vi "_wait_for_OPC.vi"(5 "Timeout in (0 = OPC timeout)":i32, 7 "Attribute":T1={"Identifier"="", "Descriptive Name"="", "Data Type"=enum."Integer 32", "Command"="", "Access"=enum."Read/Write", "Range Table"="", "Read Callback"="", "Write Callback"="", "Supported Models"="", "Instrument Options"="", "Index"=0, "OPC Wait"=FALSE, "No Status Check"=FALSE, "Cache Only"=FALSE}, 8 "error in":errorcluster caption="error in (no error)", 11 "VISA resource name":refnum<visa-resource-name>) -> (0 "error out":errorcluster, 3 "VISA resource name out":refnum<visa-resource-name>)   [LabVIEW 2020, in "Rohde&Schwarz RTx Oscilloscopes.lvlib" / "rsidr_core.lvlib"]
uses:
  rsidr_core.lvlib
  type_Attribute.ctl
  type_Attribute_Data_Type.ctl
  type_ReadWriteAccess.ctl
  type_Error_Codes.ctl
  Select Event Type.ctl
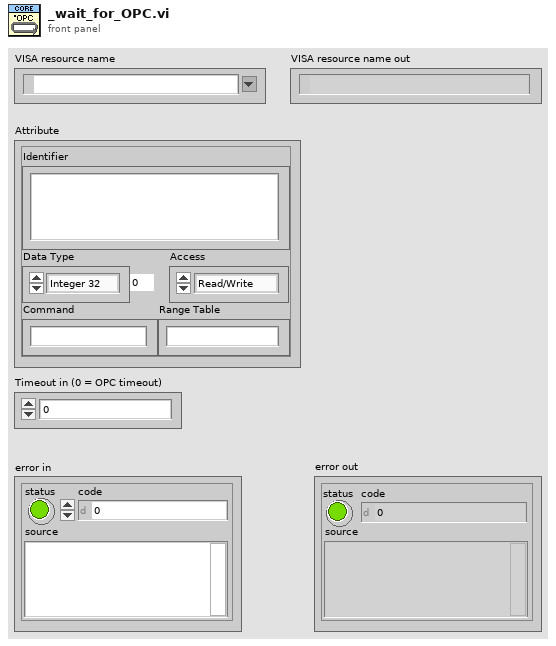
[diagram p1: front panel]
types:
  T1 = typedef "Rohde&Schwarz RTx Oscilloscopes.lvlib/rsidr_core.lvlib/type_Attribute.ctl" = cluster{"Identifier":string, "Descriptive Name":string, "Data Type":T2, "Command":string, "Access":T3, "Range Table":string, "Read Callback":string, "Write Callback":string, "Supported Models":string, "Instrument Options":string, "Index":i32, "OPC Wait":bool, "No Status Check":bool, "Cache Only":bool}
  T2 = typedef "Rohde&Schwarz RTx Oscilloscopes.lvlib/rsidr_core.lvlib/type_Attribute_Data_Type.ctl" = enum16{"Integer 32", "Double", "String", "Boolean", "None", "Integer 64", "RawString"}
  T3 = typedef "Rohde&Schwarz RTx Oscilloscopes.lvlib/rsidr_core.lvlib/type_ReadWriteAccess.ctl" = enum16{"Read Only", "Write Only", "Read/Write"}
  T4 = typedef "Rohde&Schwarz RTx Oscilloscopes.lvlib/rsidr_core.lvlib/type_Error_Codes.ctl" = enum16{"No_error", "VISA_err_ResourceNotFound", "VISA_err_Timeout", "VISA_warn_MoreDataAvailable", "RS_err_MissingCallback", "RS_err_InvalidAttribute", "RS_err_InvalidValue", "RS_err_UnknownResource", "RS_err_AlreadyInitialized", "RS_err_InstrumentStatus", "RS_err_BadRepCapName", "RS_err_TypesMismatch", "RS_err_ValueNotSupported", "RS_err_InvalidRngTable", "RS_err_IDqueryFail", "RS_err_UnexpResponse", "VISA_warn_ConfigNotLoaded", "RS_err_AttributeNotReadable", "RS_err_AttributeNotWritable", "RS_err_InstrumentType", "RS_err_InstrumentOption", "VISA_err_InvalidSize", "RS_err_ReliabilityIndicator", "VISA_warn_UnknownStatus", "VISA_warn_TermCharRead", "VISA_err_IO_error", "RS_err_FunctionNotSupported", "VISA_warn_QueueEmpty"}
  T5 = enum16{"Check error", "Don't check error", "Check error from Session"}
  T6 = typedef "Rohde&Schwarz RTx Oscilloscopes.lvlib/rsidr_core.lvlib/type_Session_Data.ctl" = cluster{"IDN string":string, "Instrument FW":string, "Instr type":string, "Instr type for err. msg.":string, "Installed Options":string[], "Ignore Error Messages":string, "Logging params":variant, "OPC Timeout":i32, "VISA Timeout":i32, "STB Poll VISA Timeout":i32, "Additional Flags":i32, "Wait Before Read":i32, "Wait Before Write":i32, "Option String Flags":i32, "IO Segment Size":i64, "VISA Access Mode":T7, "Interface Type":T8, "OPC Wait Mode":T9, "Bin Float Number  Format":T10, "Bin Integer Number Format":T11, "Simulate":bool, "VXIcapable":bool, "Duplicate Session":bool, "Add LF to Write":bool, "Logging":bool, "Fast Sweep":bool, "Query Instrument Status":bool, "Check Range":bool, "Check Options":bool, "OPC-sync Attr Writes":bool, "OPC-sync Attr Queries":bool}
  T7 = typedef "Rohde&Schwarz RTx Oscilloscopes.lvlib/rsidr_core.lvlib/type_VisaAccessMode.ctl" = u16
  T8 = typedef "Rohde&Schwarz RTx Oscilloscopes.lvlib/rsidr_core.lvlib/type_InterfaceType.ctl" = enum16{"Unknown", "GPIB", "VXI", "GPIB_VXI", "ASRL", "PXI", "TCPIP", "USB", "SOCKET"}
  T9 = typedef "Rohde&Schwarz RTx Oscilloscopes.lvlib/rsidr_core.lvlib/type_OPC_Wait_Mode.ctl" = enum16{"STBpolling", "STBpollingSlow", "STBpollingSuperSlow", "ServiceRequest", "OPCquery"}
  T10 = typedef "Rohde&Schwarz RTx Oscilloscopes.lvlib/rsidr_core.lvlib/type_Binary_Float_Number_Format.ctl" = enum16{"Float_4_Bytes_Swapped", "Float_4_Bytes", "Double_8_Bytes_Swapped", "Double_8_Bytes"}
  T11 = typedef "Rohde&Schwarz RTx Oscilloscopes.lvlib/rsidr_core.lvlib/type_Binary_Integer_Number_Format.ctl" = enum16{"Int32_4_Bytes_Swapped", "Int32_4 Bytes", "Int16_2_Bytes_Swapped", "Int16_2_Bytes"}
  T12 = typedef "Select Event Type.ctl" = u32
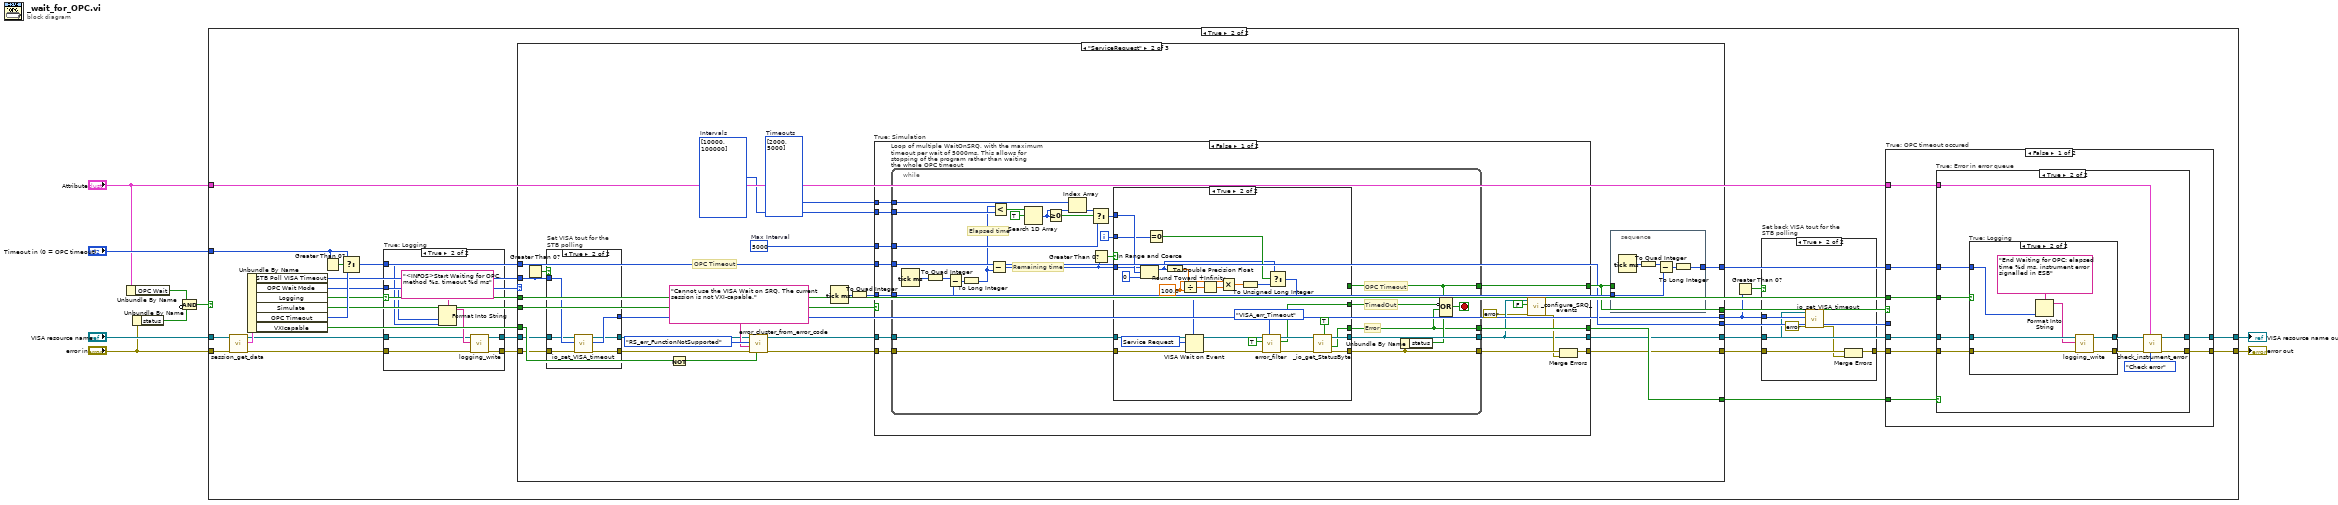
[diagram p0: block diagram]
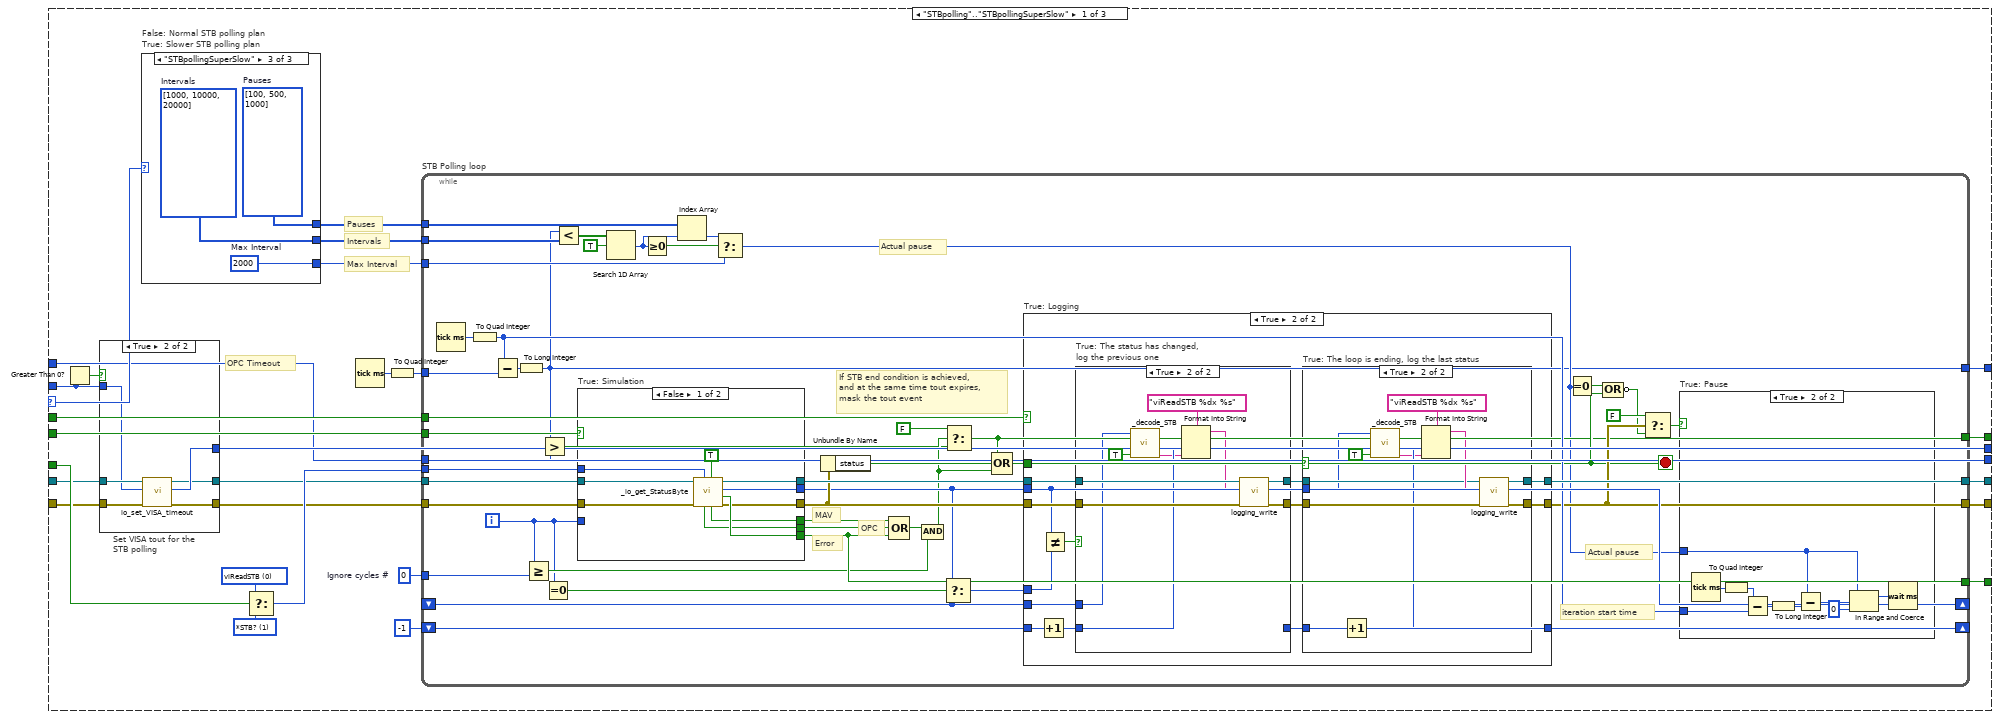
[diagram p5: hidden frame]
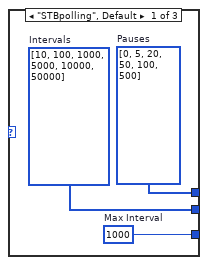
[diagram p7: hidden frame]
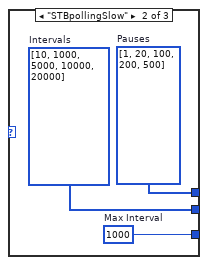
[diagram p8: hidden frame]
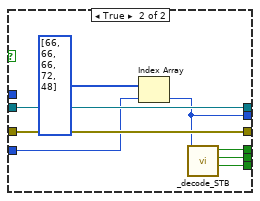
[diagram p10: hidden frame]
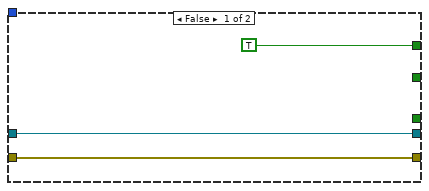
[diagram p15: hidden frame]
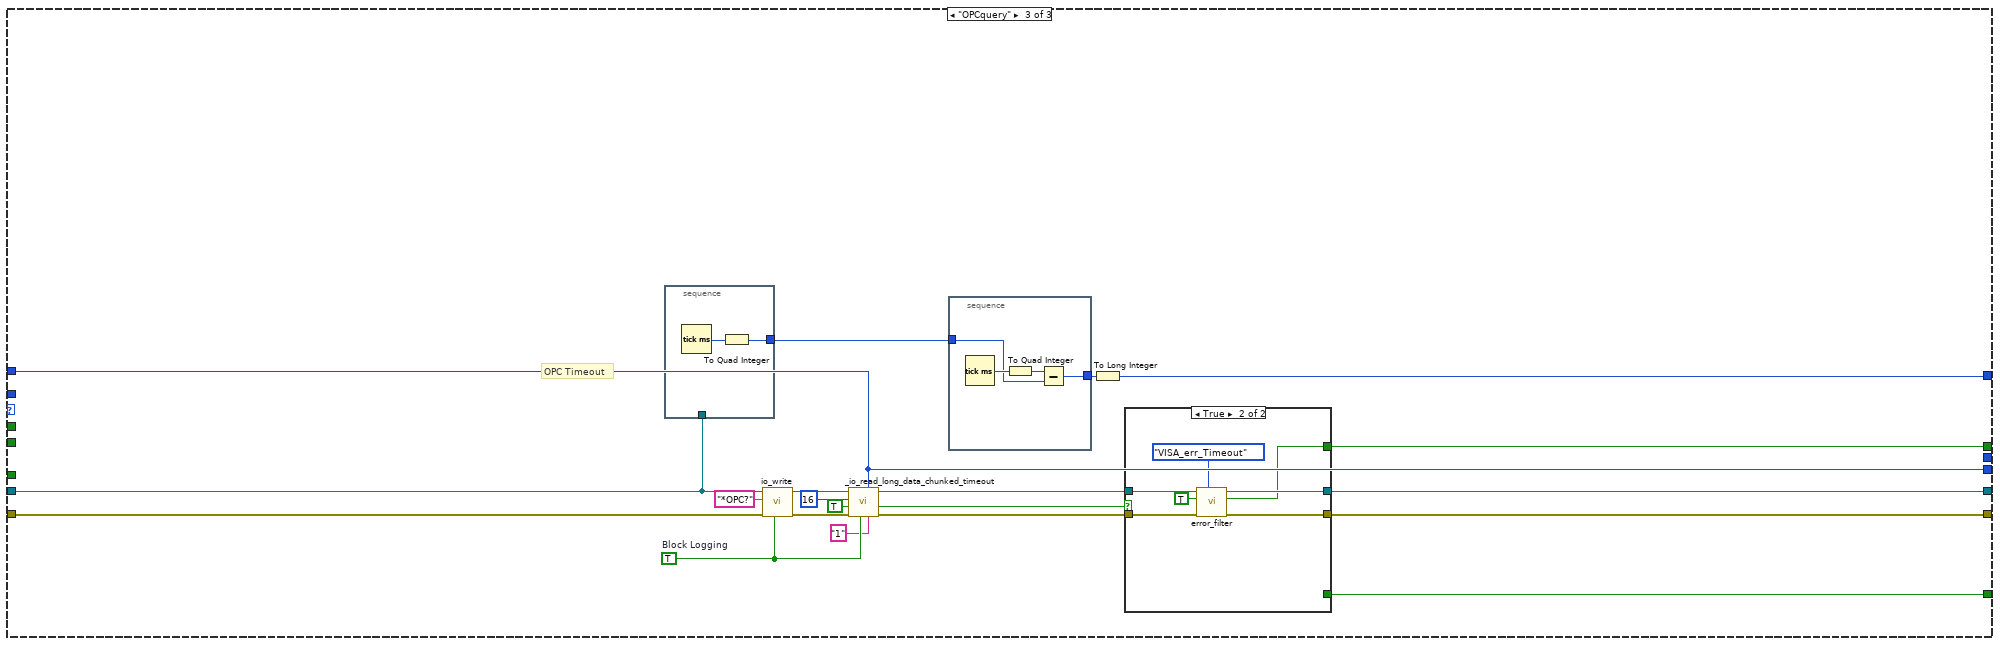
[diagram p17: hidden frame]
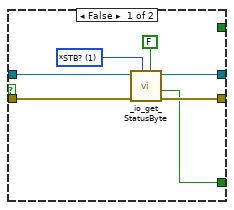
[diagram p18: hidden frame]
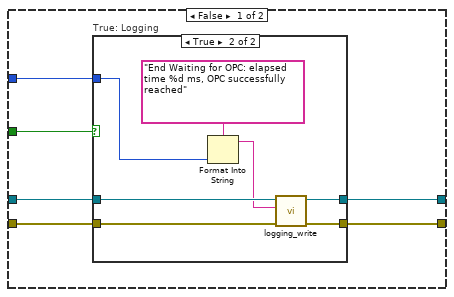
[diagram p19: hidden frame]
diagram:
  n1 = Unbundle By Name("Attribute") -> ("OPC Wait"=w2:bool)
  n2 = Unbundle By Name("error in") -> ("status"=w3:bool)
  n3 = Compound Arithmetic op=AND(w2, invert w3) -> (w1:bool)
  n4 = case shown="True" w1 {
    tunnel: "VISA resource name" -> [w11 w39]
    tunnel: "error in" -> [w10 w38]
    tunnel: [w11 w34] -> w8
    tunnel: [w10 w33] -> w9
    tunnel: "Timeout in (0 = OPC timeout)" -> [_ w27]
    tunnel: "Attribute" -> [_ w32]
    frame False {
    }
    frame True {
      n5 = call "session_get_data.vi"("error in"=w38, "VISA resource name"=w39) -> ("error out"=w25:errorcluster, "Session User Data out"=w37:T6, "VISA resource name out"=w24:refnum<visa-resource-name>)  [unwired: 6 in, 1 out]
      n6 = Unbundle By Name(w37) -> ("STB Poll VISA Timeout"=w19:i32, "OPC Wait Mode"=w20:T9, "Logging"=w21:bool, "Simulate"=w13:bool, "OPC Timeout"=w26:i32, "VXIcapable"=w30:bool)
      n7 = Greater Than 0?(x=w27) -> (x > 0?=w28:bool)
      n8 = Select(t=w27, s=w28, f=w26) -> (s? t:f=w12:i32)
      n9 = case "True: Logging" shown="True" w21 {
        tunnel: [w48 w52] -> w23
        tunnel: [w47 w51] -> w22
        tunnel: w25 -> [w48 w54]
        tunnel: w24 -> [w47 w53]
        tunnel: w20 -> [_ w50]
        tunnel: w12 -> [_ w49]
        frame False {
        }
        frame True {
          n10 = Format Into String(format string="<INFOS>Start Waiting for OPC, method %s, timeout %d ms", w50, w49) -> (resulting string=w56:string)  [unwired: 2 in, 1 out]
          n11 = call "logging_write.vi"("error in"=w54, "String to write"=w56, "VISA resource name"=w53) -> ("error out"=w52:errorcluster, "VISA resource name out"=w51:refnum<visa-resource-name>)  [unwired: 7 in]
        }
      }
      n12 = case shown="\"ServiceRequest\"" w20 {
        selector: w20 -> [w74 _ _]
        tunnel: w22 -> [w64 w226 w341]
        tunnel: [w82 w235 w333] -> w36
        tunnel: [w60 w222 w336] -> w16
        tunnel: [w81 w232 w331] -> w35
        tunnel: w13 -> [w79 w221 _]
        tunnel: w21 -> [w78 _ _]
        tunnel: [w77 w233 w335] -> w31
        tunnel: w23 -> [w65 w227 w348]
        tunnel: [w59 w219 w337] -> w18
        tunnel: w30 -> [w68 w242 _]
        tunnel: [w57 w223 w332] -> w29
        tunnel: w12 -> [w57 w223 w332]
        tunnel: w19 -> [w61 w218 _]
        tunnel: [w58 w220 _] -> w15
        frame "STBpolling".."STBpollingSuperSlow" {
          w69 = u16 1 items=["viReadSTB", "*STB?"] ("Method (viReadSTB)")
          w70 = u16 0 items=["viReadSTB", "*STB?"] ("Method (viReadSTB)")
          w76 = 0  # Ignore cycles #
          # "OPC Timeout"
          # "Pauses"
          # "Intervals"
          # "Max Interval"
          n13 = Greater Than 0?(x=w61) -> (x > 0?=w66:bool)
          n14 = case "Set VISA tout for the\nSTB polling" shown="True" w66 {
            tunnel: w65 -> [w84 w90]
            tunnel: w64 -> [w85 w89]
            tunnel: [w84 w88] -> w63
            tunnel: [w85 w87] -> w62
            tunnel: [_ w91] -> w58
            tunnel: w61 -> [_ w86]
            frame False {
            }
            frame True {
              n15 = call "io_set_VISA_timeout.vi"("error in"=w90, "VISA Timeout"=w86, "VISA resource name"=w89) -> ("error out"=w88:errorcluster, "Old VISA Timeout"=w91:u32, "VISA resource name out"=w87:refnum<visa-resource-name>)  [unwired: 6 in]
            }
          }
          n16 = case "False: Normal STB polling plan\nTrue: Slower STB polling plan" shown="\"STBpollingSuperSlow\"" w74 {
            tunnel: [w92 w95 w98] -> w72
            tunnel: [w94 w97 w100] -> w71
            tunnel: [w93 w96 w99] -> w73
            frame "STBpolling", Default {
              w93 = 1000  # Max Interval
              w92 = i32[] [0, 5, 20, 50, 100, 500]  # Pauses
              w94 = i32[] [10, 100, 1000, 5000, 10000, 50000]  # Intervals
            }
            frame "STBpollingSlow" {
              w96 = 1000  # Max Interval
              w95 = i32[] [1, 20, 100, 200, 500]  # Pauses
              w97 = i32[] [10, 1000, 5000, 10000, 20000]  # Intervals
            }
            frame "STBpollingSuperSlow" {
              w99 = 2000  # Max Interval
              w98 = i32[] [100, 500, 1000]  # Pauses
              w100 = i32[] [1000, 10000, 20000]  # Intervals
            }
          }
          n17 = Select(t=w70, s=w68, f=w69) -> (s? t:f=w67:u16)
          n18 = Tick Count (ms)() -> (millisecond timer value=w83:u32)
          n19 = To Quad Integer(1:w83) -> (0:w75:i64)
          n20 = while "STB Polling loop" {
            tunnel: [w114] -> w77
            tunnel: w75 -> [w147]
            tunnel: w57 -> [w119]
            tunnel: [w138] -> w60
            tunnel: w62 -> [w144]
            tunnel: [w143] -> w82
            tunnel: [w101] -> w81
            shift-right: [w132] -> _
            shift-left: _ -> [w131]
            tunnel: w78 -> [w130]
            shift-right: [w136] -> _
            shift-left: -1 -> [w137]
            tunnel: w79 -> [w134]
            tunnel: w76 -> [w133]
            tunnel: w67 -> [w128]
            tunnel: w63 -> [w121]
            tunnel: [w120] -> w59
            tunnel: w73 -> [w104]
            tunnel: w72 -> [w105]
            tunnel: w71 -> [w106]
            i -> [w127]
            stop <- w117 stop-if-true
            # "Actual pause"
            # "iteration start time"
            # "Actual pause"
            # "If STB end condition is achieved,\nand at the same time tout expires,\nmask the tout event"
            # "OPC"
            # "Error"
            # "MAV"
            n21 = Tick Count (ms)() -> (millisecond timer value=w125:u32)
            n22 = To Quad Integer(1:w125) -> (0:w122:i64)
            n23 = Subtract(x=w122, y=w147) -> (x-y=w107:i64)
            n24 = To Long Integer(number=w107) -> (32bit integer=w101:i32)
            n25 = Greater Or Equal?(x=w127, y=w133) -> (x >= y?=w142:bool)
            n26 = Greater?(x=w101, y=w119) -> (0:w113:bool)
            n27 = Equal To 0?(x=w127) -> (x = 0?=w126:bool)
            n28 = Less?(x=w101, y=w106) -> (x < y?=w111:bool[])
            n29 = case "True: Simulation" shown="False" w134 {
              tunnel: w121 -> [w166 w173]
              tunnel: w144 -> [w165 w174]
              tunnel: [w164 w169] -> w143
              tunnel: [w163 w171] -> w141
              tunnel: [w162 w170] -> w140
              tunnel: [w161 w174] -> w139
              tunnel: [w160 w167] -> w132
              tunnel: [w159 w173] -> w135
              tunnel: w127 -> [_ w172]
              tunnel: w128 -> [w158 _]
              frame False {
                n30 = call "_io_get_StatusByte.vi"("Block Setting of VISA Timeout for viReadSTB"=TRUE, "Method (viReadSTB)"=w158, "error in"=w166, "VISA resource name"=w165) -> ("error out"=w159:errorcluster, "Error"=w164:bool, "STB returned"=w160:u16, "VISA resource name out"=w161:refnum<visa-resource-name>, "MAV"=w162:bool, "OPC (ESB)"=w163:bool)  [unwired: 2 in]
              }
              frame True {
                n31 = Index Array(array=u16[] [66, 66, 66, 72, 48], index=w172) -> (element=w167:u16)
                n32 = call "_decode_STB.vi"("STB in"=w167) -> ("Error"=w169:bool, "OPC (ESB)"=w171:bool, "MAV"=w170:bool)  [unwired: 7 in, 1 out]
              }
            }
            n33 = Search 1D Array(1D array=w111, element=TRUE) -> (index of element=w108:i32)  [unwired: 1 in]
            n34 = Greater Or Equal To 0?(x=w108) -> (x >= 0?=w109:bool)
            n35 = Index Array(array=w105, index=w108) -> (element=w103:i32)
            n36 = Select(t=w103, s=w109, f=w104) -> (s? t:f=w102:i32)
            n37 = Unbundle By Name(w135) -> ("status"=w146:bool)
            n38 = Compound Arithmetic op=OR(w140, w141, w143) -> (w145:bool)
            n39 = Compound Arithmetic op=AND(w145, w142) -> (w115:bool)
            n40 = Select(t=w132, s=w126, f=w131) -> (s? t:f=w129:u16)
            n41 = Select(t=FALSE, s=w115, f=w113) -> (s? t:f=w114:bool)
            n42 = Compound Arithmetic op=OR(w114, w146, w115) -> (w117:bool)
            n43 = case "True: Logging" shown="True" w130 {
              tunnel: [w177 w184] -> w120
              tunnel: [w176 w183] -> w138
              tunnel: w135 -> [w177 w191]
              tunnel: w139 -> [w176 w190]
              tunnel: w137 -> [w175 w180]
              tunnel: [w175 w178] -> w136
              tunnel: w132 -> [_ w181]
              tunnel: w131 -> [_ w189]
              tunnel: w129 -> [_ w188]
              tunnel: w117 -> [_ w182]
              frame False {
              }
              frame True {
                n44 = Increment(x=w180) -> (x+1=w179:i32)
                n45 = Not Equal?(x=w181, y=w188) -> (x != y?=w187:bool)
                n46 = case "True: The status has changed,\nlog the previous one" shown="True" w187 {
                  tunnel: w191 -> [w206 w217]
                  tunnel: w190 -> [w207 w216]
                  tunnel: [w206 w215] -> w186
                  tunnel: [w207 w214] -> w185
                  tunnel: w179 -> [w205 w209]
                  tunnel: w189 -> [_ w213]
                  tunnel: [w205 _] -> w178
                  frame False {
                  }
                  frame True {
                    n47 = call "_decode_STB.vi"("Compose Summary string (F)"=TRUE ("Compose Summary String  (F)"), "STB in"=w213) -> ("Summary string"=w208:string)  [unwired: 6 in, 3 out]
                    n48 = Format Into String(format string="viReadSTB %dx %s" ("String to write"), w209, w208) -> (resulting string=w210:string)  [unwired: 2 in, 1 out]
                    n49 = call "logging_write.vi"("error in"=w217, "String to write"=w210, "VISA resource name"=w216) -> ("error out"=w215:errorcluster, "VISA resource name out"=w214:refnum<visa-resource-name>)  [unwired: 7 in]
                  }
                }
                n50 = case "True: The loop is ending, log the last status" shown="True" w182 {
                  tunnel: w186 -> [w192 w201]
                  tunnel: w185 -> [w193 w200]
                  tunnel: [w192 w199] -> w184
                  tunnel: [w193 w198] -> w183
                  tunnel: w181 -> [_ w197]
                  tunnel: w178 -> [_ w196]
                  frame False {
                  }
                  frame True {
                    n51 = Increment(x=w196) -> (x+1=w195:i32)
                    n52 = call "_decode_STB.vi"("Compose Summary string (F)"=TRUE ("Compose Summary String  (F)"), "STB in"=w197) -> ("Summary string"=w194:string)  [unwired: 6 in, 3 out]
                    n53 = Format Into String(format string="viReadSTB %dx %s" ("String to write"), w195, w194) -> (resulting string=w202:string)  [unwired: 2 in, 1 out]
                    n54 = call "logging_write.vi"("error in"=w201, "String to write"=w202, "VISA resource name"=w200) -> ("error out"=w199:errorcluster, "VISA resource name out"=w198:refnum<visa-resource-name>)  [unwired: 7 in]
                  }
                }
              }
            }
            n55 = Equal To 0?(x=w102) -> (x = 0?=w118:bool)
            n56 = Compound Arithmetic op=OR(w118, w117) -> (invert w116:bool)
            n57 = Select(t=FALSE, s=w120, f=w116) -> (s? t:f=w124:bool)
            n58 = case "True: Pause" shown="True" w124 {
              tunnel: w122 -> [_ w155]
              tunnel: w102 -> [_ w148]
              frame False {
              }
              frame True {
                n59 = Tick Count (ms)() -> (millisecond timer value=w156:u32)
                n60 = To Quad Integer(1:w156) -> (0:w152:i64)
                n61 = Subtract(x=w152, y=w155) -> (x-y=w151:i64)
                n62 = To Long Integer(number=w151) -> (32bit integer=w149:i32)
                n63 = Subtract(x=w148, y=w149) -> (x-y=w150:i32)
                n64 = In Range and Coerce(upper limit=w148, x=w150, lower limit=0) -> (coerced(x)=w153:i32)  [unwired: 1 out]
                n65 = Wait (ms)(milliseconds to wait=w153) -> ()  [unwired: 1 out]
              }
            }
          }
        }
        frame "ServiceRequest" {
          w239 = 5000  # Max Interval
          w231 = i32[] [2000, 5000]  # Timeouts
          w230 = i32[] [10000, 100000]  # Intervals
          # "OPC Timeout"
          n66 = Greater Than 0?(x=w218) -> (x > 0?=w228:bool)
          n67 = case "Set VISA tout for the\nSTB polling" shown="True" w228 {
            tunnel: w227 -> [w243 w248]
            tunnel: w226 -> [w244 w247]
            tunnel: [w243 w246] -> w225
            tunnel: [w244 w245] -> w224
            tunnel: [_ w250] -> w220
            tunnel: w218 -> [_ w249]
            frame False {
            }
            frame True {
              n68 = call "io_set_VISA_timeout.vi"("error in"=w248, "VISA Timeout"=w249, "VISA resource name"=w247) -> ("error out"=w246:errorcluster, "Old VISA Timeout"=w250:u32, "VISA resource name out"=w245:refnum<visa-resource-name>)  [unwired: 6 in]
            }
          }
          n69 = Not(x=w242) -> (.not. x?=w241:bool)
          n70 = call "error_cluster_from_error_code.vi"("Error Creation Enabled (True)"=w241, "error in"=w225, "Error Message (\"\")"="Cannot use the VISA Wait on SRQ. The current session is not VXI-capable." ("error message (\"\")"), "Error Enum in"=type_Error_Codes."RS_err_FunctionNotSupported", "VISA resource name"=w224) -> ("error out"=w237:errorcluster, "VISA resource name out"=w236:refnum<visa-resource-name>)  [unwired: 5 in]
          n71 = Tick Count (ms)() -> (millisecond timer value=w238:u32)
          n72 = To Quad Integer(1:w238) -> (0:w234:i64)
          n73 = case "True: Simulation" shown="False" w221 {
            tunnel: w231 -> [w265 _]
            tunnel: w239 -> [w264 _]
            tunnel: w230 -> [w263 _]
            tunnel: w237 -> [w262 w323]
            tunnel: w236 -> [w261 w324]
            tunnel: [w260 _] -> w235
            tunnel: w234 -> [w259 _]
            tunnel: [w258 _] -> w233
            tunnel: [w254 w323] -> w219
            tunnel: [w252 w324] -> w222
            tunnel: w223 -> [w257 _]
            frame False {
              n74 = while "Loop of multiple WaitOnSRQ, with the maximum timeout per wait of 5000ms. This allows for stopping of the program rather than waiting the whole OPC timeout" {
                tunnel: w265 -> [w287]
                tunnel: w264 -> [w275]
                tunnel: w263 -> [w286]
                tunnel: w259 -> [w280]
                tunnel: w262 -> [w285]
                tunnel: w261 -> [w284]
                tunnel: [w273] -> w255
                tunnel: [w283] -> w252
                tunnel: w257 -> [w278]
                tunnel: [w270] -> w258
                tunnel: [w268] -> w260
                i -> [w266]
                stop <- w269 stop-if-true
                # "Remaining time"
                # "Error"
                # "OPC Timeout"
                # "TimedOut"
                # "Elapsed time"
                n75 = Tick Count (ms)() -> (millisecond timer value=w282:u32)
                n76 = To Quad Integer(1:w282) -> (0:w281:i64)
                n77 = Subtract(x=w281, y=w280) -> (x-y=w279:i64)
                n78 = To Long Integer(number=w279) -> (32bit integer=w267:i32)
                n79 = Subtract(x=w278, y=w267) -> (x-y=w274:i32)
                n80 = Less?(x=w267, y=w286) -> (x < y?=w292:bool[])
                n81 = Search 1D Array(1D array=w292, element=TRUE) -> (index of element=w289:i32)  [unwired: 1 in]
                n82 = Greater Or Equal To 0?(x=w289) -> (x >= 0?=w290:bool)
                n83 = Index Array(array=w287, index=w289) -> (element=w288:i32)
                n84 = Select(t=w288, s=w290, f=w275) -> (s? t:f=w276:i32)
                n85 = Greater Than 0?(x=w274) -> (x > 0?=w277:bool)
                n86 = case shown="True" w277 {
                  tunnel: w285 -> [w295 w322]
                  tunnel: w284 -> [w293 w321]
                  tunnel: [w295 w311] -> w273
                  tunnel: [w293 w310] -> w283
                  tunnel: w274 -> [_ w319]
                  tunnel: w276 -> [_ w320]
                  tunnel: [_ w309] -> w272
                  tunnel: [TRUE _] -> w270
                  tunnel: [_ w308] -> w268
                  tunnel: w266 -> [_ w301]
                  frame False {
                  }
                  frame True {
                    w303 = 100.0 ("y")
                    w306 = T12 1073684491 items=["Service Request"=1073684491, "Trigger"=3221168138, "Clear"=1073684493, "VXI Signal"=1073684512, "VXI/VME Interrupt"=3221168161, "VXI/VME Sysfail"=1073684509, "VXI/VME Sysreset"=1073684510, "GPIB CIC"=1073684498, "GPIB Talk"=1073684499, "GPIB Listen"=1073684500, "PXI Interrupt"=1073684514, "Serial Break"=1073684515, "Serial TermChar"=1073684516, "Serial CTS"=1073684521, "Serial DSR"=1073684522, "Serial DCD"=1073684524, "Serial RI"=1073684526, "Serial Character"=1073684533, "USB Interrupt"=1073684535, "All Enabled"=1073709055] ("Event Type")
                    n87 = In Range and Coerce(upper limit=w319, x=w320, lower limit=0) -> (coerced(x)=w297:i32)  [unwired: 1 out]
                    n88 = Equal To 0?(x=w301) -> (x = 0?=w300:bool)
                    n89 = To Double Precision Float(number=w297) -> (double precision float=w299:dbl)
                    n90 = Divide(x=w299, y=w303) -> (x/y=w305:dbl)
                    n91 = Round Toward +Infinity(x=w305) -> (ceil(x): smallest int >= x=w304:dbl)
                    n92 = Multiply(x=w303, y=w304) -> (x*y=w302:dbl)
                    n93 = To Unsigned Long Integer(number=w302) -> (unsigned 32bit integer=w298:u32)
                    n94 = Select(t=w297, s=w300, f=w298) -> (s? t:f=w296:u32)
                    n95 = VISA Wait on Event(7:w296, 8:w322, 10:w306, 11:w321) -> (0:w315:errorcluster, 3:w314:refnum<visa-resource-name>)  [unwired: 1 in, 2 out]
                    n96 = call "error_filter.vi"("Error Enum in"=type_Error_Codes."VISA_err_Timeout", "error in"=w315, "Clear detected code (F)"=TRUE, "VISA resource name"=w314) -> ("error out"=w313:errorcluster, "Code Detected"=w309:bool, "VISA resource name out"=w312:refnum<visa-resource-name>)  [unwired: 5 in]
                    n97 = call "_io_get_StatusByte.vi"("Block Setting of VISA Timeout for viReadSTB"=TRUE, "error in"=w313, "VISA resource name"=w312) -> ("error out"=w311:errorcluster, "Error"=w308:bool, "VISA resource name out"=w310:refnum<visa-resource-name>)  [unwired: 3 in, 3 out]
                  }
                }
                n98 = Unbundle By Name(w273) -> ("status"=w271:bool)
                n99 = Compound Arithmetic op=OR(w270, invert w272, w268, w271) -> (w269:bool)
              }
              n100 = call "_configure_SRQ_events.vi"("error in"=errorcluster {"status"=FALSE, "code"=0, "source"=""}, "Enable"=FALSE, "VISA resource name"=w252) -> ("error out"=w253:errorcluster)  [unwired: 7 in, 1 out]
              n101 = Merge Errors(w255, w253) -> (w254:errorcluster)
            }
            frame True {
            }
          }
          n102 = stacked-sequence {
            tunnel: w234 -> [w327]
            tunnel: w233 -> [_]
            tunnel: [w325] -> w232
            frame #0 {
              n103 = Tick Count (ms)() -> (millisecond timer value=w328:u32)
              n104 = To Quad Integer(1:w328) -> (0:w329:i64)
              n105 = Subtract(x=w329, y=w327) -> (x-y=w326:i64)
              n106 = To Long Integer(number=w326) -> (32bit integer=w325:i32)
            }
          }
        }
        frame "OPCquery" {
          w344 = TRUE  # Block Logging
          # "OPC Timeout"
          n107 = stacked-sequence {
            tunnel: w341 -> [_]
            tunnel: [w364] -> w340
            frame #0 {
              n108 = Tick Count (ms)() -> (millisecond timer value=w365:u32)
              n109 = To Quad Integer(1:w365) -> (0:w364:i64)
            }
          }
          n110 = call "io_write.vi"("Block Logging (F)"=w344, "error in"=w348, "write buffer"="*OPC?", "VISA resource name"=w341) -> ("error out"=w347:errorcluster, "VISA resource name out"=w346:refnum<visa-resource-name>)  [unwired: 6 in]
          n111 = call "_io_read_long_data_chunked_timeout.vi"("Simulation read buffer (\"Simulation\")"="1" ("Simulation read buffer (\"Simulation\")"), "Timeout for chunked touts (-1: No chunked touts)"=w332, "Block Logging (F)"=w344, "error in"=w347, "Trim Response End"=TRUE ("Trim Response End (T)"), "Max segment read bytes count (65536)"=u32 16, "VISA resource name"=w346) -> ("error out"=w339:errorcluster, "TimedOut"=w334:bool, "VISA resource name out"=w338:refnum<visa-resource-name>)  [unwired: 1 in, 1 out]
          n112 = stacked-sequence {
            tunnel: [w367] -> w349
            tunnel: w340 -> [w366]
            frame #0 {
              n113 = Tick Count (ms)() -> (millisecond timer value=w368:u32)
              n114 = To Quad Integer(1:w368) -> (0:w369:i64)
              n115 = Subtract(x=w369, y=w366) -> (x-y=w367:i64)
            }
          }
          n116 = To Long Integer(number=w349) -> (32bit integer=w331:i32)
          n117 = case shown="True" w334 {
            tunnel: w339 -> [w356 w361]
            tunnel: w338 -> [w355 w360]
            tunnel: [w354 w359] -> w337
            tunnel: [w353 w358] -> w336
            tunnel: [_ w357] -> w335
            tunnel: [w352 _] -> w333
            frame False {
              w350 = u16 1 items=["viReadSTB", "*STB?"] ("Method (viReadSTB)")
              n118 = call "_io_get_StatusByte.vi"("Block Setting of VISA Timeout for viReadSTB"=FALSE, "Method (viReadSTB)"=w350, "error in"=w356, "VISA resource name"=w355) -> ("error out"=w354:errorcluster, "Error"=w352:bool, "VISA resource name out"=w353:refnum<visa-resource-name>)  [unwired: 2 in, 3 out]
            }
            frame True {
              n119 = call "error_filter.vi"("Error Enum in"=type_Error_Codes."VISA_err_Timeout", "error in"=w361, "Clear detected code (F)"=TRUE, "VISA resource name"=w360) -> ("error out"=w359:errorcluster, "Code Detected"=w357:bool, "VISA resource name out"=w358:refnum<visa-resource-name>)  [unwired: 5 in]
            }
          }
        }
      }
      n120 = Greater Than 0?(x=w15) -> (x > 0?=w14:bool)
      n121 = case "Set back VISA tout for the\nSTB polling" shown="True" w14 {
        tunnel: w18 -> [w40 w46]
        tunnel: w16 -> [_ w42]
        tunnel: [w40 w45] -> w17
        tunnel: w15 -> [_ w43]
        frame False {
        }
        frame True {
          n122 = call "io_set_VISA_timeout.vi"("error in"=errorcluster {"status"=FALSE, "code"=0, "source"=""}, "VISA Timeout"=w43, "VISA resource name"=w42) -> ("error out"=w44:errorcluster)  [unwired: 6 in, 2 out]
          n123 = Merge Errors(w46, w44) -> (w45:errorcluster)
        }
      }
      n124 = case "True: OPC timeout occured" shown="False" w31 {
        tunnel: w16 -> [w374 w419]
        tunnel: w17 -> [w376 w425]
        tunnel: [w375 w413] -> w33
        tunnel: [w373 w412] -> w34
        tunnel: w36 -> [w377 _]
        tunnel: w32 -> [w372 w414]
        tunnel: w29 -> [_ w421]
        tunnel: w21 -> [w370 w420]
        tunnel: w35 -> [w371 _]
        frame False {
          n125 = case "True: Error in error queue" shown="True" w377 {
            tunnel: w376 -> [w382 w397]
            tunnel: [w380 w402] -> w375
            tunnel: w374 -> [w383 w398]
            tunnel: [w381 w401] -> w373
            tunnel: w372 -> [_ w400]
            tunnel: w371 -> [w379 w396]
            tunnel: w370 -> [w378 w395]
            frame False {
              n126 = case "True: Logging" shown="True" w378 {
                tunnel: [w385 w390] -> w380
                tunnel: [w384 w389] -> w381
                tunnel: w382 -> [w385 w392]
                tunnel: w383 -> [w384 w391]
                tunnel: w379 -> [_ w386]
                frame False {
                }
                frame True {
                  n127 = Format Into String(format string="End Waiting for OPC: elapsed time %d ms, OPC successfully reached", w386) -> (resulting string=w388:string)  [unwired: 2 in, 1 out]
                  n128 = call "logging_write.vi"("error in"=w392, "String to write"=w388, "VISA resource name"=w391) -> ("error out"=w390:errorcluster, "VISA resource name out"=w389:refnum<visa-resource-name>)  [unwired: 7 in]
                }
              }
            }
            frame True {
              n129 = case "True: Logging" shown="True" w395 {
                tunnel: [w404 w409] -> w393
                tunnel: [w403 w408] -> w394
                tunnel: w397 -> [w404 w411]
                tunnel: w398 -> [w403 w410]
                tunnel: w396 -> [_ w405]
                frame False {
                }
                frame True {
                  n130 = Format Into String(format string="End Waiting for OPC: elapsed time %d ms, instrument error signalled in ESB", w405) -> (resulting string=w407:string)  [unwired: 2 in, 1 out]
                  n131 = call "logging_write.vi"("error in"=w411, "String to write"=w407, "VISA resource name"=w410) -> ("error out"=w409:errorcluster, "VISA resource name out"=w408:refnum<visa-resource-name>)  [unwired: 7 in]
                }
              }
              n132 = call "check_instrument_error.vi"("Mode (Check error from Session)"=T5."Check error", "Attribute"=w400, "error in"=w393, "VISA resource name"=w394) -> ("error out"=w402:errorcluster, "VISA resource name out"=w401:refnum<visa-resource-name>)  [unwired: 6 in]
            }
          }
        }
        frame True {
          n133 = Format Into String(format string="Waiting for OPC - OPC timeout error. Current OPC timeout is set to %d ms. Change it with the 'Set Timeout.vi' or 'Set OPC Timeout.vi'", w421) -> (resulting string=w423:string)  [unwired: 2 in, 1 out]
          n134 = call "_create_attribute_error.vi"("Error Elaboration (\"\")"=w423, "Attribute"=w414, "error in"=w425, "Error Enum in"=type_Error_Codes."VISA_err_Timeout" ("Error Enum in (from err to recompose)"), "VISA resource name"=w419) -> ("error out"=w422:errorcluster, "VISA resource name out"=w418:refnum<visa-resource-name>)  [unwired: 5 in]
          n135 = case "True: Logging" shown="True" w420 {
            tunnel: [w427 w432] -> w416
            tunnel: [w426 w431] -> w415
            tunnel: w422 -> [w427 w434]
            tunnel: w418 -> [w426 w433]
            tunnel: w421 -> [_ w428]
            frame False {
            }
            frame True {
              n136 = Format Into String(format string="End Waiting for OPC, timeout of %d ms reached - timeout error generated", w428) -> (resulting string=w430:string)  [unwired: 2 in, 1 out]
              n137 = call "logging_write.vi"("error in"=w434, "String to write"=w430, "VISA resource name"=w433) -> ("error out"=w432:errorcluster, "VISA resource name out"=w431:refnum<visa-resource-name>)  [unwired: 7 in]
            }
          }
          n138 = call "check_instrument_error.vi"("Attribute"=w414, "error in"=w416, "VISA resource name"=w415) -> ("error out"=w413:errorcluster, "VISA resource name out"=w412:refnum<visa-resource-name>)  [unwired: 7 in]
        }
      }
    }
  }
  "VISA resource name out" <- w8
  "error out" <- w9
